vi "State_Machine.vi"(8 "error in (no error)":errorcluster caption="entrée d'erreur (pas d'erreur)", 11 "Wait_CloseFixture en entrée":refnum<class "Wait_Voltage.lvclass">) -> (0 "error out":errorcluster caption="sortie d'erreur", 2 "Json_String":string, 3 "Wait_CloseFixture en sortie":refnum<class "Wait_Voltage.lvclass">)   [LabVIEW 2020, in "Library Test.lvlib" / "Wait_Voltage.lvclass"]
uses:
  Wait_Voltage.lvclass
  C:/Users/ngarcin/OneDrive - Altyor/Standard TB/Class/Test/Test (Default)/Test (Default).lvclass
  Instrument/Instrument (Default)/Class Instrument (Default).lvclass
  Popup/Class Popup WaitVoltage/Class Popup WaitVoltage.lvclass
  C:/Users/ngarcin/OneDrive - Altyor/Standard TB/Class/Popup/Class Popup Operator_Validation/Class Popup Operator_Validation (Default)/Class Popup Operator_Validation (Virtual).lvclass
  C:/Users/ngarcin/OneDrive - Altyor/Standard TB/Class/Popup/Class Popup (Main)/Class Popup (Main).lvclass
  Wait_Voltage.lvclass/Wait_Voltage.ctl
  Commun VI/Library Commun.lvlib
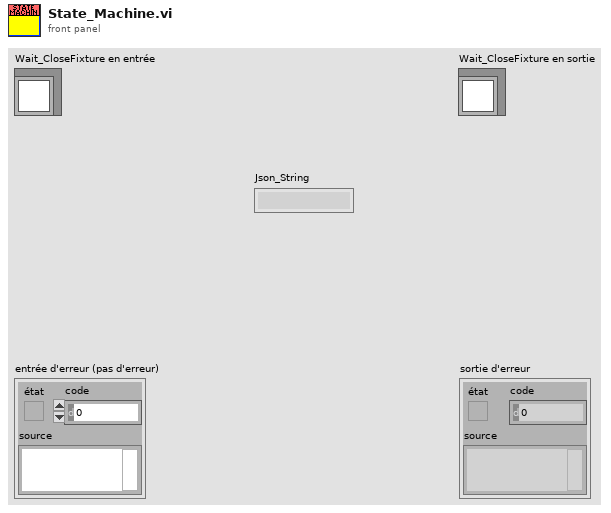
[diagram p1: front panel]
types:
  T1 = cluster{"Instrument":refnum<class "Class Instrument (Default).lvclass">, "Timeout (ms)":u64, "Value Max":dbl, "Value Min":dbl}
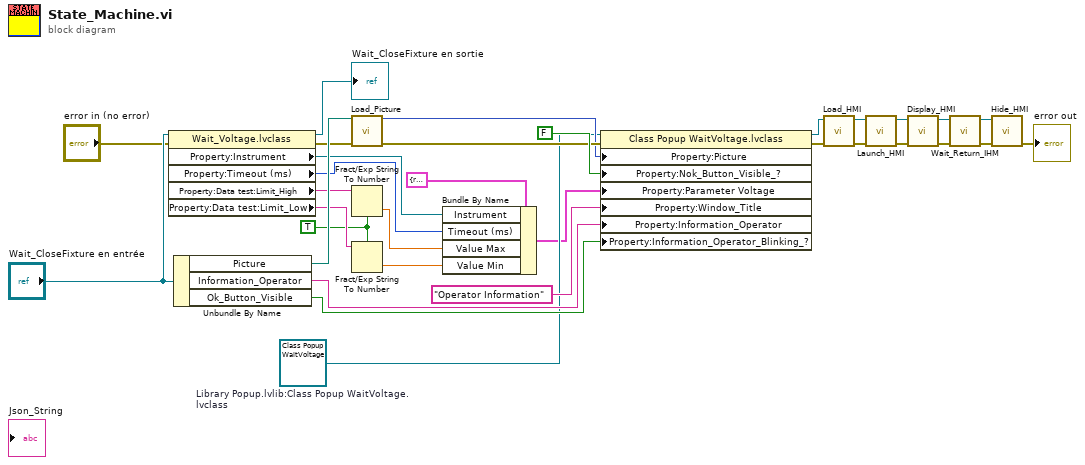
[diagram p0: block diagram]
diagram:
  w1 = TRUE ("utiliser le séparateur décimal du système (V)")
  w7 = refnum<class "Class Popup WaitVoltage.lvclass"> refnum  # Library Popup.lvlib:Class Popup WaitVoltage.lvclass
  n1 = property class="Wait_Voltage.lvclass"(reference="Wait_CloseFixture en entrée", error in="error in (no error)") -> (reference out=→"Wait_CloseFixture en sortie":refnum<class "Wait_Voltage.lvclass">, error out=w9:errorcluster, "Property:Instrument"=w11:refnum<class "Class Instrument (Default).lvclass">, "Property:Timeout (ms)"=w16:u64, "Property:Data test:Limit_High"=w4:string, "Property:Data test:Limit_Low"=w5:string)
  n2 = Unbundle By Name("Wait_CloseFixture en entrée") -> ("Picture"=w24:path, "Information_Operator"=w27:string, "Ok_Button_Visible"=w26:bool)
  n3 = call "Load_Picture.vi"("Chemin In"=w24, "error in (no error)"=w9) -> ("Img Out"=w23:picture, "error out"=w25:errorcluster)  [unwired: 11 in, 1 out]
  n4 = Fract/Exp String To Number(use system decimal point (T)=w1, string=w4) -> (number=w2:dbl)  [unwired: 2 in, 1 out]
  n5 = Fract/Exp String To Number(use system decimal point (T)=w1, string=w5) -> (number=w3:dbl)  [unwired: 2 in, 1 out]
  n6 = Bundle By Name(cluster=T1 {"Instrument"=refnum, "Timeout (ms)"=0, "Value Max"=0.0, "Value Min"=0.0} ("Parameter Voltage"), "Instrument"=w11, "Timeout (ms)"=w16, "Value Max"=w2, "Value Min"=w3) -> (w6:T1)
  n7 = property class="Class Popup WaitVoltage.lvclass"(reference=w7, error in=w25, "Property:Picture"=w23, "Property:Nok_Button_Visible_?"=FALSE ("Nok_Button_Visible_?"), "Property:Parameter Voltage"=w6, "Property:Window_Title"="Operator Information" ("Window_Title"), "Property:Information_Operator"=w27, "Property:Information_Operator_Blinking_?"=w26) -> (reference out=w31:refnum<class "Class Popup WaitVoltage.lvclass">, error out=w30:errorcluster)
  n8 = call-dynamic "Load_HMI.vi"("error in (no error)"=w30, "Class Popup (Default) en entrée"=w31) -> ("error out"=w20:errorcluster, "Class Popup (Default) en sortie"=w21:refnum<class "Class Popup WaitVoltage.lvclass">)  [unwired: 8 in]
  n9 = call-dynamic "Launch_HMI.vi"("error in (no error)"=w20, "Class Popup (Default) en entrée"=w21) -> ("error out"=w32:errorcluster, "Class Popup (Default) en sortie"=w22:refnum<class "Class Popup WaitVoltage.lvclass">)  [unwired: 8 in]
  n10 = call-dynamic "Display_HMI.vi"("error in (no error)"=w32, "Class Popup (Default) en entrée"=w22) -> ("error out"=w15:errorcluster, "Class Popup (Default) en sortie"=w12:refnum<class "Class Popup WaitVoltage.lvclass">)  [unwired: 8 in]
  n11 = call-dynamic "Wait_Return_IHM.vi"("error in (no error)"=w15, "Class Popup (Default) en entrée"=w12) -> ("error out"=w14:errorcluster, "Class Popup (Default) en sortie"=w13:refnum<class "Class Popup WaitVoltage.lvclass">)  [unwired: 8 in]
  n12 = call-dynamic "Hide_HMI.vi"("error in (no error)"=w14, "Class Popup (Default) en entrée"=w13) -> ("error out"=→"error out":errorcluster)  [unwired: 8 in, 1 out]
